vi "k_means_weighted_1D.vi"(2 "tolerance":dbl(slide)=0.12244897959183673 scale=0.0..1.0, 3 "ave":dbl[](array[numeric])=[0.9, 4.0], 4 "input and value":dbl[][](array[numeric])=[[0.1, 0.5, 1.2, 2.0, 2.4, 2.8, 3.5, 4.0, 5.0], [0.1, 2.0, 8.0, 1.3, 0.1, 0.3, 5.0, 0.4, 0.1]]) -> (0 "max":dbl[](array[numeric]), 1 "ave out":dbl[](array[numeric]))   [LabVIEW 2009]
panel:
  out "XY Graph":T1(graph)
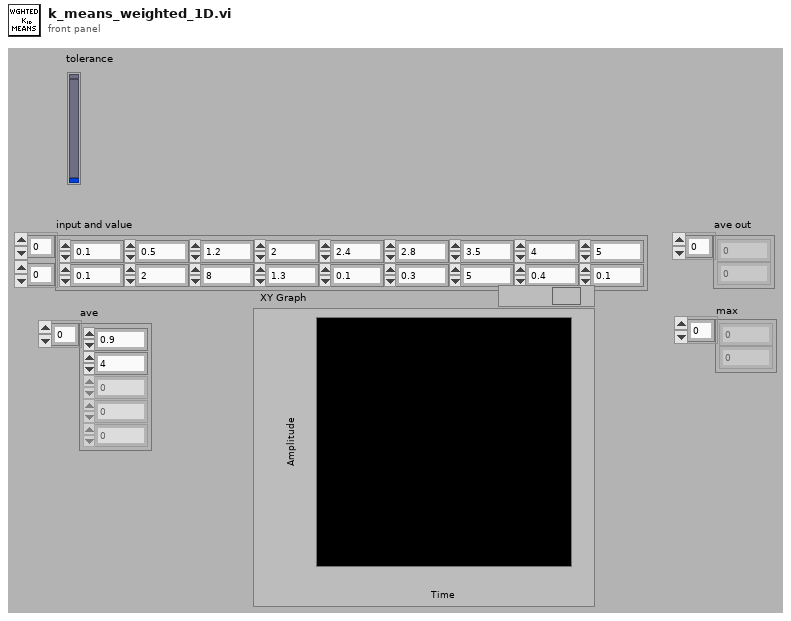
[diagram p1: front panel]
types:
  T1 = cluster{"input and value":dbl[], "input and value":dbl[]}
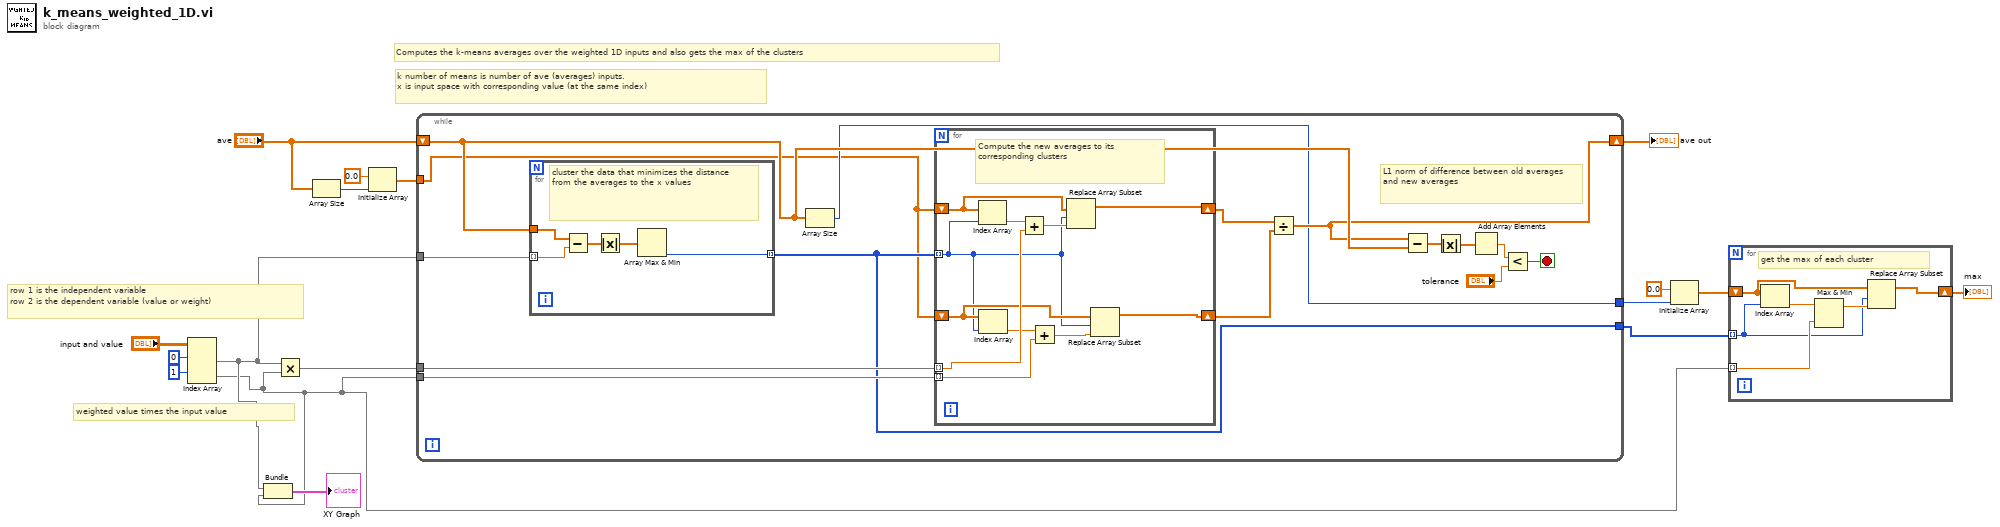
[diagram p0: block diagram]
diagram:
  # "weighted value times the input value"
  # "row 1 is the independent variable\nrow 2 is the dependent variable (value or weight)"
  # "k number of means is number of ave (averages) inputs.\nx is input space with corresponding value (at the same index)"
  # "Computes the k-means averages over the weighted 1D inputs and also gets the max of the clusters"
  n1 = Index Array(array="input and value", index (row) #1=0 ("index (row)"), index (row) #2=1 ("index (row)")) -> (element #1=w12:dbl[], element #2=w2:dbl[])  [unwired: 2 in]
  n2 = Bundle("input and value"=w12, "input and value"=w2) -> (→"XY Graph":T1)  [unwired: 1 in]
  n3 = Multiply(x=w12, y=w2) -> (x*y=w14:dbl[])
  n4 = Array Size(array="ave") -> (size(s)=w7:i32)
  n5 = Initialize Array(0.0 ("element"), w7) -> (w5:dbl[])
  n6 = while {
    tunnel: w12 -> [w32]
    tunnel: w14 -> [w31]
    shift-right: [w23] -> w13
    shift-left: "ave" -> [w30]
    tunnel: w2 -> [w22]
    tunnel: [w20] -> w3
    tunnel: [w19] -> w4
    tunnel: w5 -> [w18]
    stop <- w25 stop-if-true
    # "L1 norm of difference between old averages and new averages"
    n7 = for {
      tunnel: w32 -> [w47] mode=indexing
      tunnel: w30 -> [w48]
      tunnel: [w44] -> w20 mode=indexing
      # "cluster the data that minimizes the distance from the averages to the x values"
      n8 = Subtract(x=w48, y=w47) -> (x-y=w46:dbl[])
      n9 = Absolute Value(x=w46) -> (abs(x)=w45:dbl[])
      n10 = Array Max & Min(array=w45) -> (min index (indices)=w44:i32)  [unwired: 3 out]
    }
    n11 = Array Size(array=w30) -> (size(s)=w19:i32)
    n12 = for {
      tunnel: w20 -> [w35] mode=indexing
      shift-right: [w39] -> w24
      shift-left: w18 -> [w40]
      tunnel: w31 -> [w42] mode=indexing
      shift-right: [w33] -> w21
      shift-left: w18 -> [w36]
      tunnel: w22 -> [w37] mode=indexing
      # "Compute the new averages to its corresponding clusters"
      n13 = Index Array(array=w40, index=w35) -> (element=w43:dbl)
      n14 = Index Array(array=w36, index=w35) -> (element=w38:dbl)
      n15 = Add(x=w43, y=w42) -> (x+y=w41:dbl)
      n16 = Add(x=w38, y=w37) -> (x+y=w34:dbl)
      n17 = Replace Array Subset(array=w40, new element=w41, index=w35) -> (w39:dbl[])
      n18 = Replace Array Subset(array=w36, new element=w34, index=w35) -> (w33:dbl[])
    }
    n19 = Divide(x=w24, y=w21) -> (x/y=w23:dbl[])
    n20 = Subtract(x=w23, y=w30) -> (x-y=w29:dbl[])
    n21 = Absolute Value(x=w29) -> (abs(x)=w28:dbl[])
    n22 = Add Array Elements(numeric array=w28) -> (sum=w27:dbl)
    n23 = Less?(x=w27, y="tolerance") -> (x < y?=w25:bool)
  }
  "ave out" <- w13
  n24 = Initialize Array(0.0 ("element"), w4) -> (w10:dbl[])
  n25 = for {
    tunnel: w3 -> [w51] mode=indexing
    tunnel: w2 -> [w53] mode=indexing
    shift-right: [w49] -> w1
    shift-left: w10 -> [w50]
    # "get the max of each cluster"
    n26 = Index Array(array=w50, index=w51) -> (element=w54:dbl)
    n27 = Max & Min(x=w54, y=w53) -> (max(x,y)=w52:dbl)  [unwired: 1 out]
    n28 = Replace Array Subset(array=w50, new element=w52, index=w51) -> (w49:dbl[])
  }
  "max" <- w1
